vi "test ws client.vi"() -> ()   [LabVIEW 2016]
uses:
  http/websocket/client/websocket client.lvclass
panel:
  out "error out 2":errorcluster
  in  "send bin":bool
  in  "send txt":bool
  in  "DATA to send":string
  out "Numeric":u8=2
  out "message":string
  out "final messages":string[](array[string])
  in  "stop":bool
  out "error out":errorcluster
  in  "address":string="localhost"
  in  "port":u16=8095
  in  "url":string="dsfs"
  in  "error in":errorcluster
  in  "host header":string="sdfs"
  in  "subprotocols":string[](array[string])=["sdfs"]
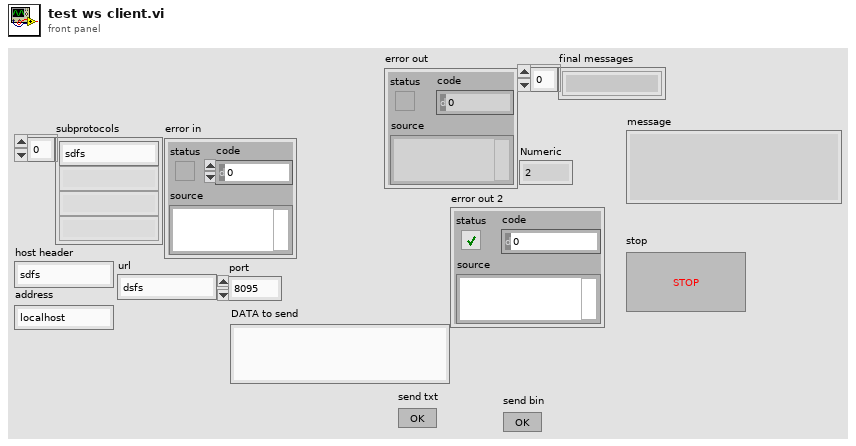
[diagram p1: front panel]
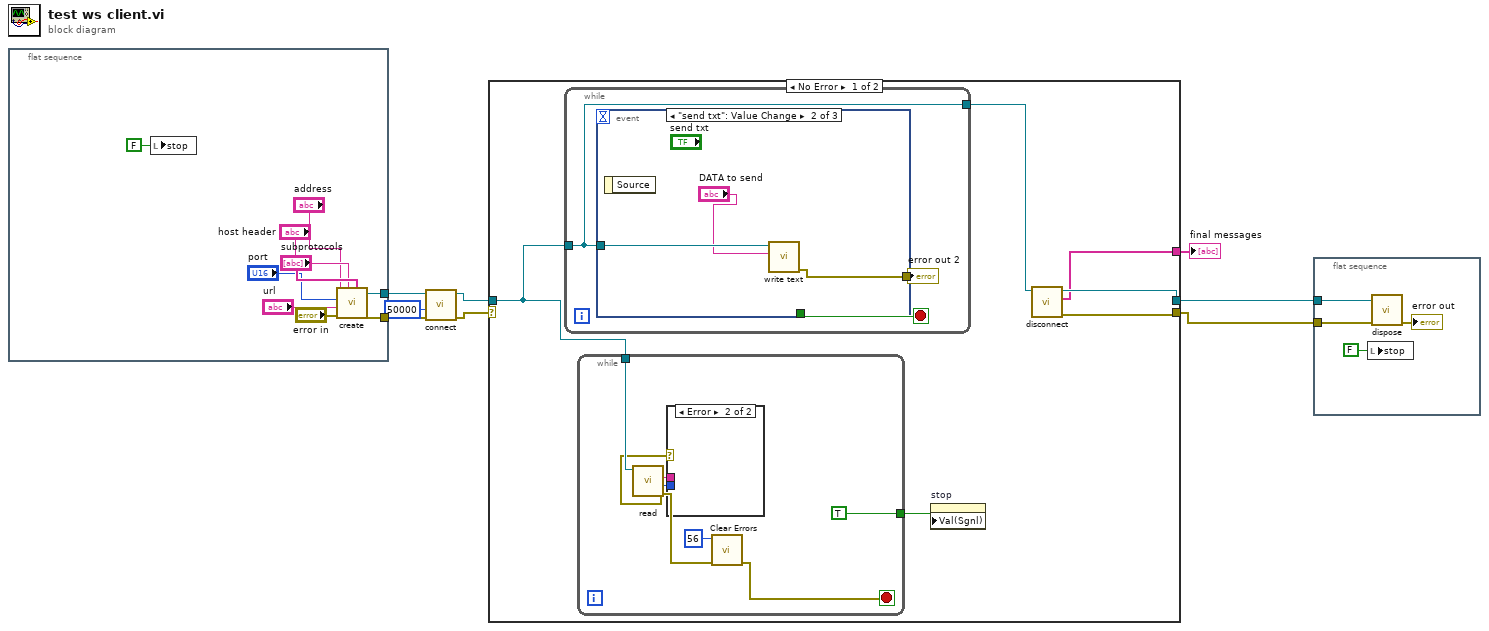
[diagram p0: block diagram]
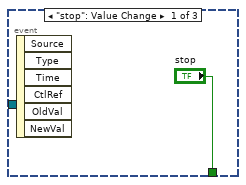
[diagram p2: hidden frame]
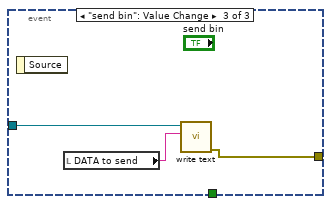
[diagram p3: hidden frame]
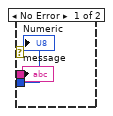
[diagram p4: hidden frame]
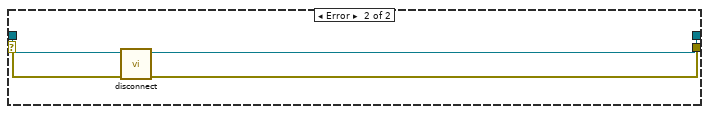
[diagram p5: hidden frame]
diagram:
  n1 = flat-sequence {
    tunnel: [w17] -> w8
    tunnel: [w16] -> w7
    frame #0 {
      n2 = local write "stop"(FALSE ("stop")) -> ()
      n3 = call "create.vi"("subprotocols"="subprotocols", "host header"="host header", "error in"="error in", "url"="url", "port"="port", "address"="address") -> ("error out"=w16:errorcluster, "websocket client out"=w17:refnum<class "websocket client.lvclass">)  [unwired: 4 in]
    }
  }
  n4 = call "connect.vi"("error in"=w7, "timeout ms (5000)"=50000, "websocket client in"=w8) -> ("error out"=w6:errorcluster, "websocket client out"=w5:refnum<class "websocket client.lvclass">)  [unwired: 7 in]
  n5 = case shown="No Error" w6 {
    selector: w6 -> [_ w46]
    tunnel: [w22 w43] -> w4
    tunnel: w5 -> [w19 w45]
    tunnel: [w23 w44] -> w3
    tunnel: [w21 _] -> w2
    frame No Error {
      n6 = while {
        tunnel: w19 -> [w24]
        tunnel: [w24] -> w18
        stop <- w26 stop-if-true
        n7 = event shown="[1] \"send txt\": Value Change" {
          selector: _ -> [_ _ _]
          dyn-events: _ -> [_ _ _]
          timeout: _ -> [_ _ _]
          tunnel: ["stop" _ _] -> w26
          tunnel: w24 -> [_ w30 w33]
          tunnel: [_ w28 w32] -> w25
          event "stop": Value Change {
            n8 = event-data() -> ()  [unwired: 1 in, 6 out]
          }
          event "send txt": Value Change {
            n9 = event-data() -> ()  [unwired: 1 in, 1 out]
            n10 = call "write text.vi"("text"="DATA to send", "websocket client in"=w30) -> ("error out"=w28:errorcluster)  [unwired: 8 in, 1 out]
          }
          event "send bin": Value Change {
            n11 = event-data() -> ()  [unwired: 1 in, 1 out]
            n12 = local read "DATA to send"() -> (w31:string)
            n13 = call "write text.vi"("text"=w31, "websocket client in"=w33) -> ("error out"=w32:errorcluster)  [unwired: 8 in, 1 out]
          }
        }
        "error out 2" <- w25
      }
      n14 = while {
        tunnel: w19 -> [w40]
        tunnel: [TRUE ("Value (Signaling)")] -> w20
        stop <- w36 stop-if-true
        n15 = call "read.vi"("websocket client in"=w40) -> ("error out"=w34:errorcluster, "Numeric"=w35:u8, "message"=w38:string)  [unwired: 7 in, 1 out]
        n16 = case shown="Error" w34 {
          tunnel: w38 -> [w42 _]
          tunnel: w35 -> [w41 _]
          frame No Error {
            "message" <- w42
            "Numeric" <- w41
          }
          frame Error {
          }
        }
        n17 = call <vilib>:"Clear Errors.vi"("error in (no error)"=w34, "specific error code to clear (0: all)"=56) -> ("error out"=w36:errorcluster)  [unwired: 4 in, 1 out]
      }
      n18 = property on="stop" class="Bool (strict)"("Val(Sgnl)"=w20) -> ()  [unwired: 2 in, 2 out]
      n19 = call "disconnect.vi"("websocket client in"=w18) -> ("error out"=w23:errorcluster, "final messages"=w21:string[], "websocket client out"=w22:refnum<class "websocket client.lvclass">)  [unwired: 8 in]
    }
    frame Error {
      n20 = call "disconnect.vi"("error in"=w46, "websocket client in"=w45) -> ("error out"=w44:errorcluster, "websocket client out"=w43:refnum<class "websocket client.lvclass">)  [unwired: 7 in, 1 out]
    }
  }
  "final messages" <- w2
  n21 = flat-sequence {
    tunnel: w4 -> [w50]
    tunnel: w3 -> [w49]
    frame #0 {
      n22 = local write "stop"(FALSE ("stop")) -> ()
      n23 = call "dispose.vi"("error in"=w49, "websocket client in"=w50) -> ("error out"=→"error out":errorcluster)  [unwired: 9 in]
    }
  }
